vi "Write ini file.vi"(6 "INI FileFullName":T1="Config.ini", 8 "error in (no error)":errorcluster, 9 "Write value":string, 10 "Name":string, 11 "section":string) -> (0 "error out":errorcluster, 1 "Boolean":bool, 2 "String value":string, 3 "DBL Value":dbl format="%#_6f", 5 "Int Value":i32)   [LabVIEW 2021, in "File RW.lvlib"]
uses:
  <userlib>/John_Lib/File/File RW.lvlib
  <userlib>/John_Lib/File/FileName.ctl
  <vilib>/Utility/config.llb/Write Key (String).vi
  <vilib>/Utility/config.llb/Read Key (String).vi
  <vilib>/Utility/config.llb/NI_LVConfig.lvlib
  <userlib>/John_Lib/TopPath/TopPath.lvlib
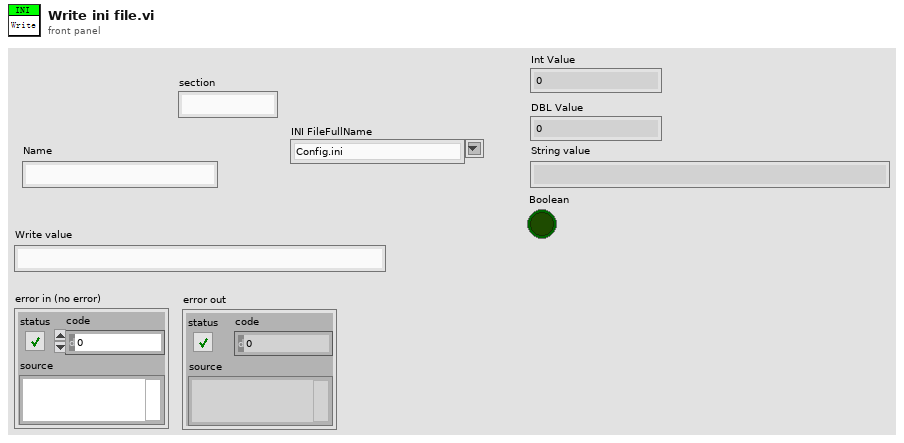
[diagram p1: front panel]
types:
  T1 = typedef "File RW.lvlib/FileName.ctl" = string
  T2 = typedef "NI_LVConfig.lvlib/Config Data RefNum.ctl" = refnum<k1>
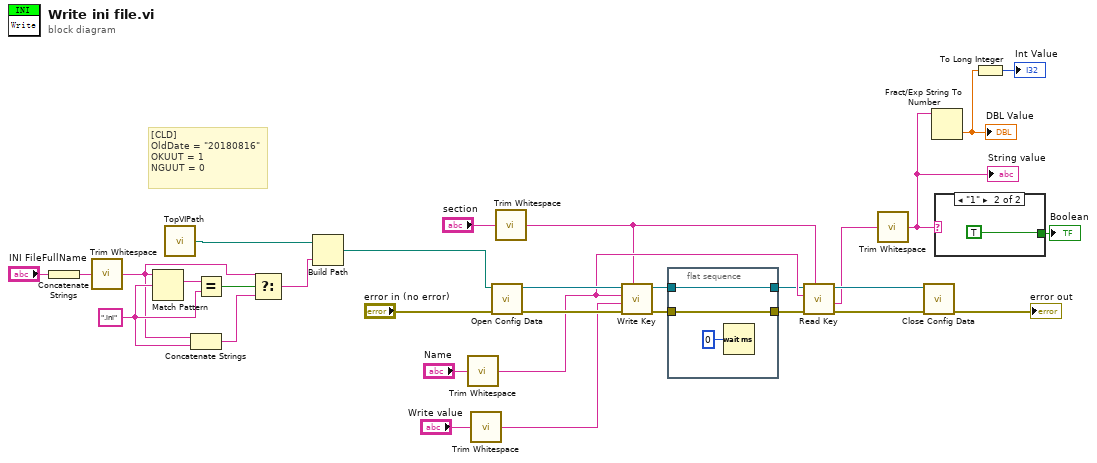
[diagram p0: block diagram]
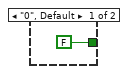
[diagram p2: hidden frame]
diagram:
  w14 = ".ini" ("regular expression")
  # "[CLD]\nOldDate = \"20180816\"\nOKUUT = 1    \nNGUUT = 0"
  n1 = Concatenate Strings("INI FileFullName") -> (w6:string)
  n2 = call <vilib>:"Trim Whitespace.vi"("string"=w6) -> ("trimmed string"=w9:string)  [unwired: 1 in]
  n3 = Match Pattern(string=w9, regular expression=w14) -> (match substring=w12:string)  [unwired: 1 in, 3 out]
  n4 = call <userlib>:"TopVIPath.vi"() -> ("ConfigFile path"=w5:path)  [unwired: 2 out]
  n5 = Concatenate Strings(w9, w14) -> (w15:string)
  n6 = Equal?(x=w12, y=w14) -> (x = y?=w13:bool)
  n7 = Select(t=w9, s=w13, f=w15) -> (s? t:f=w11:string)
  n8 = Build Path(base path=w5, name or relative path=w11) -> (appended path=w20:path)
  n9 = call <vilib>:"Trim Whitespace.vi"("string"="Name") -> ("trimmed string"=w22:string)  [unwired: 1 in]
  n10 = call <vilib>:"Trim Whitespace.vi"("string"="Write value") -> ("trimmed string"=w21:string)  [unwired: 1 in]
  n11 = call <vilib>:"Open Config Data.vi"("error in (no error)"="error in (no error)", "configuration file path"=w20) -> ("error out"=w30:errorcluster, "refnum"=w31:T2)  [unwired: 7 in, 1 out]
  n12 = call <vilib>:"Trim Whitespace.vi"("string"="section") -> ("trimmed string"=w10:string)  [unwired: 1 in]
  n13 = call-poly <vilib>:"Write Key.vi"("section"=w10, "error in (no error)"=w30, "value"=w21, "key"=w22, "refnum"=w31) -> ("error out"=w4:errorcluster, "refnum out"=w1:T2)  [unwired: 4 in, 1 out]
  n14 = flat-sequence {
    tunnel: w4 -> [w34]
    tunnel: [w34] -> w3
    tunnel: [w33] -> w2
    tunnel: w1 -> [w33]
    frame #0 {
      n15 = Wait (ms)(milliseconds to wait=u32 0) -> ()  [unwired: 1 out]
    }
  }
  n16 = call-poly <vilib>:"Read Key.vi"("section"=w10, "error in (no error)"=w3, "key"=w22, "refnum"=w2) -> ("error out"=w25:errorcluster, "value"=w18:string, "refnum out"=w24:T2)  [unwired: 4 in, 1 out]
  n17 = call <vilib>:"Trim Whitespace.vi"("string"=w18) -> ("trimmed string"=w8:string)  [unwired: 1 in]
  "String value" <- w8
  n18 = call <vilib>:"Close Config Data.vi"("error in (no error)"=w25, "refnum"=w24) -> ("error out"=→"error out":errorcluster)  [unwired: 8 in, 1 out]
  n19 = Fract/Exp String To Number(string=w8) -> (number=w17:dbl)  [unwired: 3 in, 1 out]
  "DBL Value" <- w17
  n20 = case shown="\"1\"" w8 {
    tunnel: [FALSE ("Boolean") TRUE ("Boolean")] -> w19
    frame "0", Default {
    }
    frame "1" {
    }
  }
  "Boolean" <- w19
  n21 = To Long Integer(number=w17) -> (32bit integer=→"Int Value":i32)
